vi "LSMcontroller_v58.vi"() -> ()   [LabVIEW 2015] (continued)
                        n3600 = call "waveformsDObuffer.vi"("DO wf in"=w272, "command"="set") -> ()  [unwired: 1 out]
                        n3601 = local write "Total Camera Frames"(w273) -> ()
                        n3602 = local read "wavdet"() -> (w270:bool)
                        n3603 = case shown="True" w270 {
                          tunnel: w269 -> [_ w288]
                          frame False {
                          }
                          frame True {
                            n3604 = local write "# of frames"(w288) -> ()
                          }
                        }
                      }
                    }
                  }
                  frame #6 {
                    w295 = FALSE ("addAO")
                    # "set signaling boolean to false"
                    n3605 = local read "finite samples"() -> (w296:bool)
                    n3606 = local read "continuous"() -> (w297:bool)
                    n3607 = local read "wavdet"() -> (w298:bool)
                    n3608 = call "2pparameters.vi"("command"="get") -> ("params out"=w301:T12)  [unwired: 1 in]
                    n3609 = Bundle By Name(cluster=w301, "finite"=w296, "cont"=w297, "wavdet"=w298) -> (w299:T12)
                    n3610 = local write "addAO"(w295) -> ()
                    n3611 = property on="Add AO wave" class="Bool (strict)"("Val(Sgnl)"=w295) -> ()  [unwired: 2 in, 2 out]
                    n3612 = call "2pparameters.vi"("Params in"=w299, "command"="set") -> ()  [unwired: 1 out]
                  }
                }
              }
            }
          }
          event "AO channels": Value Change {
            n3613 = event-data() -> ()  [unwired: 1 in, 6 out]
            n3614 = local read "AO channels"() -> (w303:u32)
            n3615 = call "2pparameters.vi"("command"="get") -> ("params out"=w305:T12)  [unwired: 1 in]
            n3616 = Unbundle By Name(w305) -> ("aAO"=w304:u32[])
            n3617 = Search 1D Array(1D array=w304, element=w303) -> (index of element=w307:i32)  [unwired: 1 in]
            n3618 = Equal?(x=w307, y=-1.0) -> (x = y?=w308:bool)
            n3619 = case shown="False" w308 {
              tunnel: w307 -> [w310 _]
              frame False {
                n3620 = call "waveformparamsv2.vi"("command"="get") -> ("Params out"=w317:T16)  [unwired: 4 in, 2 out]
                n3621 = Unbundle By Name(w317) -> ("AO parameters"=w316:T17)
                n3622 = Index Array(array=w316, index=w310) -> (element=w333:T18)
                n3623 = Unbundle By Name(w333) -> ("AOtab"=w314:dbl, "Repeats"=w332:dbl, "Cycles"=w331:dbl, "Start amplitude (V)"=w330:dbl, "Baseline (V)"=w329:dbl, "Step size (V)"=w328:dbl, "DC (%)"=w327:dbl, "Sampling frequency (Hz)"=w326:dbl, "Period (ms)"=w325:dbl, "Offset (V)"=w324:dbl, "Amplitude (V)"=w323:dbl, "Frequency"=w322:dbl, "Tri Repeats"=w321:dbl, "phase shift (ms)"=w320:dbl, "Pulses"=w319:dbl, "Tri phase"=w315:dbl, "padding value"=w311:dbl, "Matlab wave file"=w312:path)
                n3624 = To Unsigned Long Integer(number=w314) -> (unsigned 32bit integer=w313:u32)
                n3625 = local write "Build analog waveform tabs"(w313) -> ()
                n3626 = local write "Matlab waveform path"(w312) -> ()
                n3627 = local write "phase shift (ms)"(w320) -> ()
                n3628 = local write "Repeats"(w332) -> ()
                n3629 = local write "Cycles"(w331) -> ()
                n3630 = local write "Amplitude (V)"(w323) -> ()
                n3631 = local write "Matlab padding value"(w311) -> ()
                n3632 = local write "Tri padding value"(w311) -> ()
                n3633 = local write "Start amplitude (V)"(w330) -> ()
                n3634 = local write "Tri Phase (s)"(w315) -> ()
                n3635 = local write "Period (ms)"(w325) -> ()
                n3636 = local write "Tri Repeats"(w321) -> ()
                n3637 = local write "Offset (V)"(w324) -> ()
                n3638 = local write "Frequency"(w322) -> ()
                n3639 = local write "Pulses"(w319) -> ()
                n3640 = local write "padding value"(w311) -> ()
                n3641 = local write "Sampling rate \ncurrent wf"(w326) -> ()
                n3642 = local write "Baseline (V)"(w329) -> ()
                n3643 = local write "Step size (V)"(w328) -> ()
                n3644 = local write "DC (%)"(w327) -> ()
                "Numeric" <- w310
              }
              frame True {
              }
            }
          }
          event "Rem AO wave": Value Change {
            n3645 = event-data() -> ("NewVal"=w334:bool)  [unwired: 1 in, 5 out]
            n3646 = case shown="True" w334 {
              frame False {
              }
              frame True {
                n3647 = stacked-sequence {
                  seq-local: [_ _ w440 _ _ _ _] -> [_ _ _ _ w460 w463 _]
                  frame #0 {
                    n3648 = local read "Measurement"() -> (w335:T5)
                    n3649 = case shown="\"X-Y-t movie\", Default" w335 {
                      frame "X-Y-t movie", Default {
                        n3650 = local read "avpp"() -> (w356:i32)
                        n3651 = local read "Angle ref"() -> (w355:dbl)
                        n3652 = local read "ROI Type"() -> (w354:u16)
                        n3653 = local read "xpixels ref"() -> (w351:i32)
                        n3654 = local read "Vx-min ref"() -> (w350:dbl)
                        n3655 = local read "Vx-max ref"() -> (w349:dbl)
                        n3656 = local read "ypixels ref"() -> (w347:i32)
                        n3657 = local read "Vy-min ref"() -> (w348:dbl)
                        n3658 = local read "Vy-max ref"() -> (w344:dbl)
                        n3659 = local read "Sampling rate"() -> (w338:dbl)
                        n3660 = local read "finite samples"() -> (w339:bool)
                        n3661 = local read "continuous"() -> (w342:bool)
                        n3662 = local read "wavdet"() -> (w343:bool)
                        n3663 = local read "# of frames"() -> (w341:i32)
                        n3664 = local read "maxbufferAI"() -> (w340:i32)
                        n3665 = local read "Override AI buffer"() -> (w336:bool)
                        n3666 = call "2pparameters.vi"("command"="get") -> ("params out"=w353:T12)  [unwired: 1 in]
                        n3667 = Bundle By Name(cluster=w353, "type"="X-Y-t movie", "avpp"=w356, "Angle Img"=w355, "Xpixels Img"=w351, "Vx-min Img"=w350, "VX-max Img"=w349, "Ypixels Img"=w347, "Vy-min Img"=w348, "Vy-max Img"=w344, "srate"=w338, "srate Img"=w338, "finite"=w339, "cont"=w342, "wavdet"=w343, "measpoints"=w341, "maxbufferAI"=w340, "Drawing Mode"=w354, "Vz-reset"=0.0, "AIoverride"=w336) -> (w345:T12)
                        n3668 = call "2pparameters.vi"("Params in"=w345, "command"="set") -> ()  [unwired: 1 out]
                      }
                      frame "X-Y-Z stack" {
                        n3669 = call "2pparameters.vi"("command"="get") -> ("params out"=w360:T12)  [unwired: 1 in]
                        n3670 = Bundle By Name(cluster=w360, "type"="X-Y-Z stack") -> (w358:T12)
                        n3671 = call "2pparameters.vi"("Params in"=w358, "command"="set") -> ()  [unwired: 1 out]
                      }
                      frame "Lifetime (scan)" {
                        n3672 = call "2pparameters.vi"("command"="get") -> ("params out"=w365:T12)  [unwired: 1 in]
                        n3673 = Bundle By Name(cluster=w365, "type"="Lifetime (scan)") -> (w363:T12)
                        n3674 = call "2pparameters.vi"("Params in"=w363, "command"="set") -> ()  [unwired: 1 out]
                      }
                      frame "Lifetime (contour)" {
                        n3675 = local read "Vy-min draw"() -> (w375:dbl)
                        n3676 = local read "Vy-max draw"() -> (w374:dbl)
                        n3677 = local read "Vx-min draw"() -> (w377:dbl)
                        n3678 = local read "Vx-max draw"() -> (w376:dbl)
                        n3679 = local read "xpixels ref"() -> (w373:i32)
                        n3680 = local read "ypixels ref"() -> (w372:i32)
                        n3681 = local read "ROI Type"() -> (w371:u16)
                        n3682 = local read "srateAODOtt"() -> (w382:dbl)
                        n3683 = local read "# of frames"() -> (w387:i32)
                        n3684 = local read "refreshtime"() -> (w379:dbl)
                        n3685 = local read "Pel"() -> (w370:dbl)
                        n3686 = local read "bin"() -> (w385:dbl)
                        n3687 = local read "Override AI buffer"() -> (w368:bool)
                        n3688 = local read "finite samples"() -> (w394:bool)
                        n3689 = local read "srateAODOtt"() -> (w381:dbl)
                        n3690 = local read "srateAODOtt"() -> (w388:dbl)
                        n3691 = local read "continuous"() -> (w393:bool)
                        n3692 = local read "Angle ref"() -> (w378:dbl)
                        n3693 = local read "wavdet"() -> (w395:bool)
                        n3694 = local read "Vx-ref"() -> (w390:dbl)
                        n3695 = local read "Vy-ref"() -> (w392:dbl)
                        n3696 = local read "avpp"() -> (w391:i32)
                        n3697 = call "tt_timeandsamples.vi"("bin"=w385, "refreshtime"=w379, "srateAODOtt"=w382, "tot#ofsamples"=w387) -> ("refreshrate"=w383:dbl, "refreshbuffer"=w384:i32, "timetracecycles"=w389:i32)  [unwired: 5 in]
                        n3698 = local read "bin"() -> (w386:dbl)
                        n3699 = call "2pparameters.vi"("command"="get") -> ("params out"=w398:T12)  [unwired: 1 in]
                        n3700 = Bundle By Name(cluster=w398, "Drawing Mode"=w371, "measpoints"=w387, "tt_cycles"=w389, "refreshbuffer"=w384, "refreshrate"=w383, "Vx-ref"=w390, "Vy-ref"=w392, "srate"=w381, "finite"=w394, "cont"=w393, "wavdet"=w395, "avpp"=w391, "srateAODO"=w388, "bufferAI"=w384, "bin"=w386, "Angle Img"=w378, "Vxminref"=w377, "Vxmaxref"=w376, "Vyminref"=w375, "Vymaxref"=w374, "Xpixels Img"=w373, "Ypixels Img"=w372, "Pel"=w370, "Vz-reset"=0.0, "AIoverride"=w368, "type"="Lifetime (contour)") -> (w396:T12)
                        n3701 = Reciprocal(x=w383) -> (1/x=w380:dbl)
                        n3702 = local write "refreshtime"(w380) -> ()
                        n3703 = call "2pparameters.vi"("Params in"=w396, "command"="set") -> ()  [unwired: 1 out]
                      }
                      frame "X-Y-Z-t movie" {
                      }
                      frame "linescan" {
                      }
                      frame "Timetrace" {
                        n3704 = local read "Vy-min draw"() -> (w408:dbl)
                        n3705 = local read "Vy-max draw"() -> (w407:dbl)
                        n3706 = local read "Vx-min draw"() -> (w410:dbl)
                        n3707 = local read "Vx-max draw"() -> (w409:dbl)
                        n3708 = local read "xpixels ref"() -> (w406:i32)
                        n3709 = local read "ypixels ref"() -> (w405:i32)
                        n3710 = local read "ROI Type"() -> (w404:u16)
                        n3711 = local read "srateAODOtt"() -> (w415:dbl)
                        n3712 = local read "# of frames"() -> (w420:i32)
                        n3713 = local read "refreshtime"() -> (w412:dbl)
                        n3714 = local read "Pel"() -> (w403:dbl)
                        n3715 = local read "bin"() -> (w418:dbl)
                        n3716 = local read "Override AI buffer"() -> (w401:bool)
                        n3717 = local read "finite samples"() -> (w427:bool)
                        n3718 = local read "srateAODOtt"() -> (w414:dbl)
                        n3719 = local read "srateAODOtt"() -> (w421:dbl)
                        n3720 = local read "continuous"() -> (w426:bool)
                        n3721 = local read "Angle ref"() -> (w411:dbl)
                        n3722 = local read "wavdet"() -> (w428:bool)
                        n3723 = local read "Vx-ref"() -> (w423:dbl)
                        n3724 = local read "Vy-ref"() -> (w425:dbl)
                        n3725 = local read "avpp"() -> (w424:i32)
                        n3726 = call "tt_timeandsamples.vi"("bin"=w418, "refreshtime"=w412, "srateAODOtt"=w415, "tot#ofsamples"=w420) -> ("refreshrate"=w416:dbl, "refreshbuffer"=w417:i32, "timetracecycles"=w422:i32)  [unwired: 5 in]
                        n3727 = local read "bin"() -> (w419:dbl)
                        n3728 = call "2pparameters.vi"("command"="get") -> ("params out"=w431:T12)  [unwired: 1 in]
                        n3729 = Bundle By Name(cluster=w431, "Drawing Mode"=w404, "measpoints"=w420, "tt_cycles"=w422, "refreshbuffer"=w417, "refreshrate"=w416, "Vx-ref"=w423, "Vy-ref"=w425, "srate"=w414, "finite"=w427, "cont"=w426, "wavdet"=w428, "avpp"=w424, "srateAODO"=w421, "bufferAI"=w417, "bin"=w419, "Angle Img"=w411, "Vxminref"=w410, "Vxmaxref"=w409, "Vyminref"=w408, "Vymaxref"=w407, "Xpixels Img"=w406, "Ypixels Img"=w405, "Pel"=w403, "Vz-reset"=0.0, "AIoverride"=w401, "type"="Timetrace") -> (w429:T12)
                        n3730 = Reciprocal(x=w416) -> (1/x=w413:dbl)
                        n3731 = local write "refreshtime"(w413) -> ()
                        n3732 = call "2pparameters.vi"("Params in"=w429, "command"="set") -> ()  [unwired: 1 out]
                      }
                      frame "Lifetime (point)" {
                      }
                    }
                  }
                  frame #1 {
                    w434 = FALSE ("wavdet")
                    n3733 = call "2pparameters.vi"("command"="get") -> ("params out"=w438:T12)  [unwired: 1 in]
                    n3734 = Bundle By Name(cluster=w438, "finite"=w434, "cont"=w434, "wavdet"=TRUE) -> (w435:T12)
                    n3735 = call "2pparameters.vi"("Params in"=w435, "command"="set") -> ()  [unwired: 1 out]
                  }
                  frame #2 {
                    # "remove channel from numbers array"
                    n3736 = local read "AO channels"() -> (w445:u32)
                    n3737 = call "2pparameters.vi"("command"="get") -> ("params out"=w443:T12)  [unwired: 1 in]
                    n3738 = in-place {
                      in-place-border: w445 -> [w451]
                      in-place-border: [w448] -> w446
                      in-place-border: [w447] -> w440
                      n3739 = in-place-cluster #50(w443) -> ("aAO"=w450:u32[])
                      n3740 = call "remove channel from active arrayv2.vi"("line array in"=w450, "line to remove"=w451) -> ("line array out"=w449:u32[], "removal"=w448:bool, "index"=w447:i32)
                      n3741 = in-place-cluster #50("aAO"=w449) -> (w441:T12)
                    }
                    n3742 = local write "remAO"(w446) -> ()
                    n3743 = call "2pparameters.vi"("Params in"=w441, "command"="set") -> ()  [unwired: 1 out]
                  }
                  frame #3 {
                    n3744 = local read "remAO"() -> (w452:bool)
                    n3745 = case shown="True" w452 {
                      frame False {
                      }
                      frame True {
                        n3746 = call "Used AO lines.vi"() -> ("used AO names"=w456:string[], "used AO lines"=w458:tag[])  [unwired: 2 in]
                        n3747 = control-ref of="Analog Lines Plot"() -> (w457:refnum<vi>)
                        n3748 = control-ref of="Digital Lines Plot"() -> (w455:refnum<vi>)
                        n3749 = call "Used DO lines.vi"() -> ("used DO names"=w454:string[], "used DO lines"=w453:tag[])  [unwired: 2 in]
                        n3750 = local write "Analog Used Lines"(w458) -> ()
                        n3751 = local write "Analog Used Names"(w456) -> ()
                        n3752 = local write "Digital Used Lines"(w453) -> ()
                        n3753 = local write "Digital Used Names"(w454) -> ()
                        n3754 = call "prepDOWaveplot.vi"("DigitalGraph in"=w455, "used DO names"=w454) -> ()  [unwired: 1 in]
                        n3755 = call "prepAOWaveplot.vi"("WaveformGraph in"=w457, "Analog Used Names"=w456) -> ()  [unwired: 1 in]
                      }
                    }
                  }
                  frame #4 {
                    n3756 = local read "remAO"() -> (w459:bool)
                    n3757 = case shown="True" w459 {
                      tunnel: w460 -> [_ w461]
                      frame False {
                      }
                      frame True {
                        n3758 = call "waveformparamsv2.vi"("command"="rem AO", "index"=w461) -> ()  [unwired: 3 in, 3 out]
                      }
                    }
                  }
                  frame #5 {
                    n3759 = local read "remAO"() -> (w464:bool)
                    n3760 = case shown="True" w464 {
                      tunnel: w463 -> [_ w483]
                      frame False {
                      }
                      frame True {
                        n3761 = local read "Meastab"() -> (w468:enum32{"X-Y Image", "Linescan", "Timetrace"})
                        n3762 = property on="refwf" class="Ring (strict)"() -> ("RingText.Text"=w471:string)  [unwired: 2 in, 2 out]
                        n3763 = case shown="\"Timetrace\"" w468 {
                          tunnel: [w484 w485] -> w467
                          frame "X-Y Image", Default {
                            n3764 = local read "Sampling rate"() -> (w484:dbl)
                          }
                          frame "Timetrace" {
                            n3765 = local read "srateAODOtt"() -> (w485:dbl)
                          }
                        }
                        n3766 = call "waveformsAObuffer.vi"("command"="get") -> ("AO wf out"=w480:waveform(dbl)[])  [unwired: 1 in]
                        n3767 = call "waveformsDObuffer.vi"("command"="get") -> ("DO wf out"=w477:digitalwaveform[])  [unwired: 1 in]
                        n3768 = Delete From Array(array=w480, length=1, index=w483) -> (array with subset deleted=w472:waveform(dbl)[])  [unwired: 1 out]
                        n3769 = call "correctwaveformsizetemp.vi"("new sampling frequency (Hz)"=w467, "start"=FALSE, "reference waveforms to"=w471, "Analog waveforms in"=w472, "stop"=FALSE, "Digital waveforms in"=w477) -> ("analog wf out"=w475:waveform(dbl)[], "Digital wf out"=w473:digitalwaveform[], "measpoints"=w469:i32)
                        n3770 = local write "Analog Lines Plot"(w475) -> ()
                        n3771 = call "GetNumCamFramesv2.vi"("Digital Waveform Graph"=w473) -> ("Numeric"=w474:i32)  [unwired: 10 in]
                        n3772 = local write "Digital Lines Plot"(w473) -> ()
                        n3773 = call "waveformsAObuffer.vi"("AO wf in"=w475, "command"="set") -> ()  [unwired: 1 out]
                        n3774 = call "waveformsDObuffer.vi"("DO wf in"=w473, "command"="set") -> ()  [unwired: 1 out]
                        n3775 = local read "wavdet"() -> (w470:bool)
                        n3776 = local write "Total Camera Frames"(w474) -> ()
                        n3777 = case shown="True" w470 {
                          tunnel: w469 -> [_ w486]
                          frame False {
                          }
                          frame True {
                            n3778 = local write "# of frames"(w486) -> ()
                          }
                        }
                      }
                    }
                  }
                  frame #6 {
                    w487 = FALSE ("remAO")
                    n3779 = local read "finite samples"() -> (w488:bool)
                    n3780 = local read "continuous"() -> (w489:bool)
                    n3781 = local read "wavdet"() -> (w490:bool)
                    n3782 = call "2pparameters.vi"("command"="get") -> ("params out"=w493:T12)  [unwired: 1 in]
                    n3783 = Bundle By Name(cluster=w493, "finite"=w488, "cont"=w489, "wavdet"=w490) -> (w491:T12)
                    n3784 = local write "remAO"(w487) -> ()
                    n3785 = property on="Rem AO wave" class="Bool (strict)"("Val(Sgnl)"=w487) -> ()  [unwired: 2 in, 2 out]
                    n3786 = call "2pparameters.vi"("Params in"=w491, "command"="set") -> ()  [unwired: 1 out]
                  }
                }
              }
            }
          }
          event "Add DO wave": Value Change {
            n3787 = event-data() -> ("NewVal"=w495:bool)  [unwired: 1 in, 5 out]
            n3788 = case shown="True" w495 {
              frame False {
              }
              frame True {
                n3789 = stacked-sequence {
                  seq-local: [_ _ _ _ _ w655 _ _] -> [_ _ _ _ _ _ w670 _]
                  frame #0 {
                    n3790 = local read "Measurement"() -> (w496:T5)
                    n3791 = case shown="\"X-Y-t movie\", Default" w496 {
                      frame "X-Y-t movie", Default {
                        n3792 = local read "avpp"() -> (w517:i32)
                        n3793 = local read "Angle ref"() -> (w516:dbl)
                        n3794 = local read "ROI Type"() -> (w515:u16)
                        n3795 = local read "xpixels ref"() -> (w512:i32)
                        n3796 = local read "Vx-min ref"() -> (w511:dbl)
                        n3797 = local read "Vx-max ref"() -> (w510:dbl)
                        n3798 = local read "ypixels ref"() -> (w508:i32)
                        n3799 = local read "Vy-min ref"() -> (w509:dbl)
                        n3800 = local read "Vy-max ref"() -> (w505:dbl)
                        n3801 = local read "Sampling rate"() -> (w499:dbl)
                        n3802 = local read "finite samples"() -> (w500:bool)
                        n3803 = local read "continuous"() -> (w503:bool)
                        n3804 = local read "wavdet"() -> (w504:bool)
                        n3805 = local read "# of frames"() -> (w502:i32)
                        n3806 = local read "maxbufferAI"() -> (w501:i32)
                        n3807 = local read "Override AI buffer"() -> (w497:bool)
                        n3808 = call "2pparameters.vi"("command"="get") -> ("params out"=w514:T12)  [unwired: 1 in]
                        n3809 = Bundle By Name(cluster=w514, "type"="X-Y-t movie", "avpp"=w517, "Angle Img"=w516, "Xpixels Img"=w512, "Vx-min Img"=w511, "VX-max Img"=w510, "Ypixels Img"=w508, "Vy-min Img"=w509, "Vy-max Img"=w505, "srate"=w499, "srate Img"=w499, "finite"=w500, "cont"=w503, "wavdet"=w504, "measpoints"=w502, "maxbufferAI"=w501, "Drawing Mode"=w515, "Vz-reset"=0.0, "AIoverride"=w497) -> (w506:T12)
                        n3810 = call "2pparameters.vi"("Params in"=w506, "command"="set") -> ()  [unwired: 1 out]
                      }
                      frame "X-Y-Z stack" {
                        n3811 = call "2pparameters.vi"("command"="get") -> ("params out"=w521:T12)  [unwired: 1 in]
                        n3812 = Bundle By Name(cluster=w521, "type"="X-Y-Z stack") -> (w519:T12)
                        n3813 = call "2pparameters.vi"("Params in"=w519, "command"="set") -> ()  [unwired: 1 out]
                      }
                      frame "Lifetime (scan)" {
                        n3814 = call "2pparameters.vi"("command"="get") -> ("params out"=w526:T12)  [unwired: 1 in]
                        n3815 = Bundle By Name(cluster=w526, "type"="Lifetime (scan)") -> (w524:T12)
                        n3816 = call "2pparameters.vi"("Params in"=w524, "command"="set") -> ()  [unwired: 1 out]
                      }
                      frame "Lifetime (contour)" {
                        n3817 = local read "Vy-min draw"() -> (w536:dbl)
                        n3818 = local read "Vy-max draw"() -> (w535:dbl)
                        n3819 = local read "Vx-min draw"() -> (w538:dbl)
                        n3820 = local read "Vx-max draw"() -> (w537:dbl)
                        n3821 = local read "xpixels ref"() -> (w534:i32)
                        n3822 = local read "ypixels ref"() -> (w533:i32)
                        n3823 = local read "ROI Type"() -> (w532:u16)
                        n3824 = local read "srateAODOtt"() -> (w543:dbl)
                        n3825 = local read "# of frames"() -> (w548:i32)
                        n3826 = local read "refreshtime"() -> (w540:dbl)
                        n3827 = local read "Pel"() -> (w531:dbl)
                        n3828 = local read "bin"() -> (w546:dbl)
                        n3829 = local read "Override AI buffer"() -> (w529:bool)
                        n3830 = local read "finite samples"() -> (w555:bool)
                        n3831 = local read "srateAODOtt"() -> (w542:dbl)
                        n3832 = local read "srateAODOtt"() -> (w549:dbl)
                        n3833 = local read "continuous"() -> (w554:bool)
                        n3834 = local read "Angle ref"() -> (w539:dbl)
                        n3835 = local read "wavdet"() -> (w556:bool)
                        n3836 = local read "Vx-ref"() -> (w551:dbl)
                        n3837 = local read "Vy-ref"() -> (w553:dbl)
                        n3838 = local read "avpp"() -> (w552:i32)
                        n3839 = call "tt_timeandsamples.vi"("bin"=w546, "refreshtime"=w540, "srateAODOtt"=w543, "tot#ofsamples"=w548) -> ("refreshrate"=w544:dbl, "refreshbuffer"=w545:i32, "timetracecycles"=w550:i32)  [unwired: 5 in]
                        n3840 = local read "bin"() -> (w547:dbl)
                        n3841 = call "2pparameters.vi"("command"="get") -> ("params out"=w559:T12)  [unwired: 1 in]
                        n3842 = Bundle By Name(cluster=w559, "Drawing Mode"=w532, "measpoints"=w548, "tt_cycles"=w550, "refreshbuffer"=w545, "refreshrate"=w544, "Vx-ref"=w551, "Vy-ref"=w553, "srate"=w542, "finite"=w555, "cont"=w554, "wavdet"=w556, "avpp"=w552, "srateAODO"=w549, "bufferAI"=w545, "bin"=w547, "Angle Img"=w539, "Vxminref"=w538, "Vxmaxref"=w537, "Vyminref"=w536, "Vymaxref"=w535, "Xpixels Img"=w534, "Ypixels Img"=w533, "Pel"=w531, "Vz-reset"=0.0, "AIoverride"=w529, "type"="Lifetime (contour)") -> (w557:T12)
                        n3843 = Reciprocal(x=w544) -> (1/x=w541:dbl)
                        n3844 = local write "refreshtime"(w541) -> ()
                        n3845 = call "2pparameters.vi"("Params in"=w557, "command"="set") -> ()  [unwired: 1 out]
                      }
                      frame "X-Y-Z-t movie" {
                      }
                      frame "linescan" {
                      }
                      frame "Timetrace" {
                        n3846 = local read "Vy-min draw"() -> (w569:dbl)
                        n3847 = local read "Vy-max draw"() -> (w568:dbl)
                        n3848 = local read "Vx-min draw"() -> (w571:dbl)
                        n3849 = local read "Vx-max draw"() -> (w570:dbl)
                        n3850 = local read "xpixels ref"() -> (w567:i32)
                        n3851 = local read "ypixels ref"() -> (w566:i32)
                        n3852 = local read "ROI Type"() -> (w565:u16)
                        n3853 = local read "srateAODOtt"() -> (w576:dbl)
                        n3854 = local read "# of frames"() -> (w581:i32)
                        n3855 = local read "refreshtime"() -> (w573:dbl)
                        n3856 = local read "Pel"() -> (w564:dbl)
                        n3857 = local read "bin"() -> (w579:dbl)
                        n3858 = local read "Override AI buffer"() -> (w562:bool)
                        n3859 = local read "finite samples"() -> (w588:bool)
                        n3860 = local read "srateAODOtt"() -> (w575:dbl)
                        n3861 = local read "srateAODOtt"() -> (w582:dbl)
                        n3862 = local read "continuous"() -> (w587:bool)
                        n3863 = local read "Angle ref"() -> (w572:dbl)
                        n3864 = local read "wavdet"() -> (w589:bool)
                        n3865 = local read "Vx-ref"() -> (w584:dbl)
                        n3866 = local read "Vy-ref"() -> (w586:dbl)
                        n3867 = local read "avpp"() -> (w585:i32)
                        n3868 = call "tt_timeandsamples.vi"("bin"=w579, "refreshtime"=w573, "srateAODOtt"=w576, "tot#ofsamples"=w581) -> ("refreshrate"=w577:dbl, "refreshbuffer"=w578:i32, "timetracecycles"=w583:i32)  [unwired: 5 in]
                        n3869 = local read "bin"() -> (w580:dbl)
                        n3870 = call "2pparameters.vi"("command"="get") -> ("params out"=w592:T12)  [unwired: 1 in]
                        n3871 = Bundle By Name(cluster=w592, "Drawing Mode"=w565, "measpoints"=w581, "tt_cycles"=w583, "refreshbuffer"=w578, "refreshrate"=w577, "Vx-ref"=w584, "Vy-ref"=w586, "srate"=w575, "finite"=w588, "cont"=w587, "wavdet"=w589, "avpp"=w585, "srateAODO"=w582, "bufferAI"=w578, "bin"=w580, "Angle Img"=w572, "Vxminref"=w571, "Vxmaxref"=w570, "Vyminref"=w569, "Vymaxref"=w568, "Xpixels Img"=w567, "Ypixels Img"=w566, "Pel"=w564, "Vz-reset"=0.0, "AIoverride"=w562, "type"="Timetrace") -> (w590:T12)
                        n3872 = Reciprocal(x=w577) -> (1/x=w574:dbl)
                        n3873 = local write "refreshtime"(w574) -> ()
                        n3874 = call "2pparameters.vi"("Params in"=w590, "command"="set") -> ()  [unwired: 1 out]
                      }
                      frame "Lifetime (point)" {
                      }
                    }
                  }
                  frame #1 {
                    w595 = FALSE ("wavdet")
                    n3875 = call "2pparameters.vi"("command"="get") -> ("params out"=w599:T12)  [unwired: 1 in]
                    n3876 = Bundle By Name(cluster=w599, "finite"=w595, "cont"=w595, "wavdet"=TRUE) -> (w596:T12)
                    n3877 = call "2pparameters.vi"("Params in"=w596, "command"="set") -> ()  [unwired: 1 out]
                  }
                  frame #2 {
                    n3878 = local read "DO channels"() -> (w606:u16)
                    n3879 = call "2pparameters.vi"("command"="get") -> ("params out"=w604:T12)  [unwired: 1 in]
                    n3880 = in-place {
                      in-place-border: w606 -> [w610]
                      in-place-border: [w607] -> w601
                      n3881 = in-place-cluster #51(w604) -> ("aDO"=w609:u32[])
                      n3882 = call "add channel to active arrayv2.vi"("line array in"=w609, "line to add"=w610) -> ("line array out"=w608:u32[], "addition"=w607:bool)  [unwired: 1 out]
                      n3883 = in-place-cluster #51("aDO"=w608) -> (w602:T12)
                    }
                    n3884 = local write "addDO"(w601) -> ()
                    n3885 = call "2pparameters.vi"("Params in"=w602, "command"="set") -> ()  [unwired: 1 out]
                  }
                  frame #3 {
                    n3886 = local read "addDO"() -> (w611:bool)
                    n3887 = case shown="True" w611 {
                      frame False {
                      }
                      frame True {
                        n3888 = call "Used AO lines.vi"() -> ("used AO names"=w615:string[], "used AO lines"=w617:tag[])  [unwired: 2 in]
                        n3889 = control-ref of="Analog Lines Plot"() -> (w616:refnum<vi>)
                        n3890 = control-ref of="Digital Lines Plot"() -> (w614:refnum<vi>)
                        n3891 = call "Used DO lines.vi"() -> ("used DO names"=w613:string[], "used DO lines"=w612:tag[])  [unwired: 2 in]
                        n3892 = local write "Analog Used Lines"(w617) -> ()
                        n3893 = local write "Analog Used Names"(w615) -> ()
                        n3894 = local write "Digital Used Lines"(w612) -> ()
                        n3895 = local write "Digital Used Names"(w613) -> ()
                        n3896 = call "prepDOWaveplot.vi"("DigitalGraph in"=w614, "used DO names"=w613) -> ()  [unwired: 1 in]
                        n3897 = call "prepAOWaveplot.vi"("WaveformGraph in"=w616, "Analog Used Names"=w615) -> ()  [unwired: 1 in]
                      }
                    }
                  }
                  frame #4 {
                    n3898 = local read "addDO"() -> (w618:bool)
                    n3899 = case shown="True" w618 {
                      frame False {
                      }
                      frame True {
                        n3900 = local read "Build digital waveform tabs"() -> (w619:enum32{"Simple", "Matlab"})
                        n3901 = case shown="\"Matlab\"" w619 {
                          frame "Simple", Default {
                            n3902 = local read "Meastab"() -> (w621:enum32{"X-Y Image", "Linescan", "Timetrace"})
                            n3903 = call "waveformparamsv2.vi"("command"="get") -> ("Params out"=w635:T16)  [unwired: 4 in, 2 out]
                            n3904 = case shown="\"Timetrace\"" w621 {
                              tunnel: [w637 w638] -> w620
                              frame "X-Y Image", Default {
                                n3905 = local read "Sampling rate"() -> (w637:dbl)
                              }
                              frame "Timetrace" {
                                n3906 = local read "srateAODOtt"() -> (w638:dbl)
                              }
                            }
                            n3907 = Unbundle By Name(w635) -> ("DO parameters"=w633:T19)
                            n3908 = local read "Digital padding value"() -> (w624:dbl)
                            n3909 = local read "Digital time offset (s)"() -> (w625:dbl)
                            n3910 = local read "Digital phase (s)"() -> (w627:dbl)
                            n3911 = local read "Digital Freq (Hz)"() -> (w626:dbl)
                            n3912 = local read "Digital DC (%)"() -> (w628:dbl)
                            n3913 = Index Array(array=w633, index=0) -> (element=w632:T20)
                            n3914 = Bundle By Name(cluster=w632, "Digital DC (%)"=w628, "Digital phase"=w627, "Digital Freq (Hz)"=w626, "Sampling frequency (Hz)"=w620, "Digital time offset (s)"=w625, "padding value"=w624, "matlab wave file"=path "", "DOtab"=0.0) -> (w630:T20)
                            n3915 = Build Array(w630) -> (w629:T19)
                            n3916 = call "waveformparamsv2.vi"("command"="add DO", "add DO"=w629) -> ()  [unwired: 3 in, 3 out]
                          }
                          frame "Matlab" {
                            w642 = 0.0 ("DOtab")
                            n3917 = local read "Meastab"() -> (w640:enum32{"X-Y Image", "Linescan", "Timetrace"})
                            n3918 = call "waveformparamsv2.vi"("command"="get") -> ("Params out"=w651:T16)  [unwired: 4 in, 2 out]
                            n3919 = case shown="\"Timetrace\"" w640 {
                              tunnel: [w653 w654] -> w639
                              frame "X-Y Image", Default {
                                n3920 = local read "Sampling rate"() -> (w653:dbl)
                              }
                              frame "Timetrace" {
                                n3921 = local read "srateAODOtt"() -> (w654:dbl)
                              }
                            }
                            n3922 = Unbundle By Name(w651) -> ("DO parameters"=w649:T19)
                            n3923 = local read "Matlab waveform path DO"() -> (w641:path)
                            n3924 = local read "Matlab padding value DO"() -> (w644:dbl)
                            n3925 = Index Array(array=w649, index=0) -> (element=w648:T20)
                            n3926 = Bundle By Name(cluster=w648, "Digital DC (%)"=w642, "Digital phase"=w642, "Digital Freq (Hz)"=w642, "Sampling frequency (Hz)"=w639, "Digital time offset (s)"=w642, "padding value"=w644, "matlab wave file"=w641, "DOtab"=1.0) -> (w646:T20)
                            n3927 = Build Array(w646) -> (w645:T19)
                            n3928 = call "waveformparamsv2.vi"("command"="add DO", "add DO"=w645) -> ()  [unwired: 3 in, 3 out]
                          }
                        }
                      }
                    }
                  }
                  frame #5 {
                    n3929 = local read "addDO"() -> (w656:bool)
                    n3930 = case shown="True" w656 {
                      tunnel: [_ w657] -> w655
                      frame False {
                      }
                      frame True {
                        n3931 = property on="refwf" class="Ring (strict)"() -> ("RingText.Text"=w662:string)  [unwired: 2 in, 2 out]
                        n3932 = call "waveformsDObuffer.vi"("command"="get") -> ("DO wf out"=w661:digitalwaveform[])  [unwired: 1 in]
                        n3933 = call "waveformsAObuffer.vi"("command"="get") -> ("AO wf out"=w659:waveform(dbl)[])  [unwired: 1 in]
                        n3934 = call "referfencesize.vi"("Digital waveforms in"=w661, "Analog waveforms in"=w659, "reference waveforms to"=w662) -> ("number of samples"=w657:i32)  [unwired: 2 in]
                      }
                    }
                  }
                  frame #6 {
                    n3935 = local read "Build digital waveform tabs"() -> (w673:enum32{"Simple", "Matlab"})
                    n3936 = call "waveformparamsv2.vi"("command"="get last DO") -> ("last DO"=w672:T20)  [unwired: 4 in, 2 out]
                    n3937 = local read "Meastab"() -> (w666:enum32{"X-Y Image", "Linescan", "Timetrace"})
                    n3938 = call "waveformsDObuffer.vi"("command"="get") -> ("DO wf out"=w671:digitalwaveform[])  [unwired: 1 in]
                    n3939 = case shown="\"Simple\", Default" w673 {
                      tunnel: w672 -> [w690 w692]
                      tunnel: w670 -> [w689 _]
                      tunnel: [w688 w691] -> w669
                      frame "Simple", Default {
                        n3940 = call "simple digital from wf params.vi"("waveform params"=w690, "number of samples"=w689) -> ("digital waveform"=w688:digitalwaveform)
                      }
                      frame "Matlab" {
                        n3941 = call "matlabDOwffromparam.vi"("waveform params"=w692) -> ("digital waveform"=w691:digitalwaveform)
                      }
                    }
                    n3942 = property on="refwf" class="Ring (strict)"() -> ("RingText.Text"=w676:string)  [unwired: 2 in, 2 out]
                    n3943 = case shown="\"Timetrace\"" w666 {
                      tunnel: [w685 w686] -> w665
                      frame "X-Y Image", Default {
                        n3944 = local read "Sampling rate"() -> (w685:dbl)
                      }
                      frame "Timetrace" {
                        n3945 = local read "srateAODOtt"() -> (w686:dbl)
                      }
                    }
                    n3946 = call "waveformsAObuffer.vi"("command"="get") -> ("AO wf out"=w684:waveform(dbl)[])  [unwired: 1 in]
                    n3947 = Build Array (concatenate)(w671, w669) -> (w675:digitalwaveform[])
                    n3948 = call "correctwaveformsizetemp.vi"("new sampling frequency (Hz)"=w665, "start"=FALSE, "reference waveforms to"=w676, "Analog waveforms in"=w684, "stop"=FALSE, "Digital waveforms in"=w675) -> ("analog wf out"=w679:waveform(dbl)[], "Digital wf out"=w677:digitalwaveform[], "measpoints"=w667:i32)
                    n3949 = local write "Analog Lines Plot"(w679) -> ()
                    n3950 = call "GetNumCamFramesv2.vi"("Digital Waveform Graph"=w677) -> ("Numeric"=w678:i32)  [unwired: 10 in]
                    n3951 = local write "Digital Lines Plot"(w677) -> ()
                    n3952 = call "waveformsAObuffer.vi"("AO wf in"=w679, "command"="set") -> ()  [unwired: 1 out]
                    n3953 = call "waveformsDObuffer.vi"("DO wf in"=w677, "command"="set") -> ()  [unwired: 1 out]
                    n3954 = local write "Total Camera Frames"(w678) -> ()
                    n3955 = local read "wavdet"() -> (w668:bool)
                    n3956 = case shown="True" w668 {
                      tunnel: w667 -> [_ w687]
                      frame False {
                      }
                      frame True {
                        n3957 = local write "# of frames"(w687) -> ()
                      }
                    }
                  }
                  frame #7 {
                    w693 = FALSE ("addAO")
                    n3958 = local read "finite samples"() -> (w694:bool)
                    n3959 = local read "continuous"() -> (w695:bool)
                    n3960 = local read "wavdet"() -> (w696:bool)
                    n3961 = call "2pparameters.vi"("command"="get") -> ("params out"=w699:T12)  [unwired: 1 in]
                    n3962 = Bundle By Name(cluster=w699, "finite"=w694, "cont"=w695, "wavdet"=w696) -> (w697:T12)
                    n3963 = call "2pparameters.vi"("Params in"=w697, "command"="set") -> ()  [unwired: 1 out]
                    n3964 = local write "addDO"(w693) -> ()
                    n3965 = property on="Add DO wave" class="Bool (strict)"("Val(Sgnl)"=w693) -> ()  [unwired: 2 in, 2 out]
                  }
                }
              }
            }
          }
          event "DO channels": Value Change {
            n3966 = event-data() -> ()  [unwired: 1 in, 6 out]
            n3967 = local read "DO channels"() -> (w703:u16)
            n3968 = call "2pparameters.vi"("command"="get") -> ("params out"=w705:T12)  [unwired: 1 in]
            n3969 = Unbundle By Name(w705) -> ("aDO"=w704:u32[])
            n3970 = Search 1D Array(1D array=w704, element=w703) -> (index of element=w702:i32)  [unwired: 1 in]
            n3971 = Equal?(x=w702, y=-1.0) -> (x = y?=w701:bool)
            n3972 = case shown="False" w701 {
              tunnel: w702 -> [w720 _]
              frame False {
                n3973 = call "waveformparamsv2.vi"("command"="get") -> ("Params out"=w715:T16)  [unwired: 4 in, 2 out]
                n3974 = Unbundle By Name(w715) -> ("DO parameters"=w713:T19)
                n3975 = Index Array(array=w713, index=w720) -> (element=w719:T20)
                n3976 = Unbundle By Name(w719) -> ("Digital DC (%)"=w718:dbl, "Digital phase"=w717:dbl, "Digital Freq (Hz)"=w716:dbl, "Sampling frequency (Hz)"=w708:dbl, "Digital time offset (s)"=w712:dbl, "padding value"=w711:dbl, "matlab wave file"=w710:path, "DOtab"=w709:dbl)
                n3977 = local write "Build digital waveform tabs"(w709) -> ()
                n3978 = local write "Digital DC (%)"(w718) -> ()
                n3979 = local write "Matlab waveform path DO"(w710) -> ()
                n3980 = local write "Digital time offset (s)"(w712) -> ()
                n3981 = local write "Matlab padding value DO"(w711) -> ()
                n3982 = local write "Digital padding value"(w711) -> ()
                n3983 = local write "Sampling rate \ncurrent wf"(w708) -> ()
                n3984 = local write "Digital Freq (Hz)"(w716) -> ()
                n3985 = local write "Digital phase (s)"(w717) -> ()
              }
              frame True {
              }
            }
          }
          event "Rem DO wave": Value Change {
            n3986 = event-data() -> ("NewVal"=w721:bool)  [unwired: 1 in, 5 out]
            n3987 = case shown="True" w721 {
              frame False {
              }
              frame True {
                n3988 = stacked-sequence {
                  seq-local: [_ _ w827 _ _ _ _] -> [_ _ _ _ w846 w857 _]
                  frame #0 {
                    n3989 = local read "Measurement"() -> (w722:T5)
                    n3990 = case shown="\"linescan\"" w722 {
                      frame "X-Y-t movie", Default {
                        n3991 = local read "avpp"() -> (w743:i32)
                        n3992 = local read "Angle ref"() -> (w742:dbl)
                        n3993 = local read "ROI Type"() -> (w741:u16)
                        n3994 = local read "xpixels ref"() -> (w738:i32)
                        n3995 = local read "Vx-min ref"() -> (w737:dbl)
                        n3996 = local read "Vx-max ref"() -> (w736:dbl)
                        n3997 = local read "ypixels ref"() -> (w734:i32)
                        n3998 = local read "Vy-min ref"() -> (w735:dbl)
                        n3999 = local read "Vy-max ref"() -> (w731:dbl)
                        n4000 = local read "Sampling rate"() -> (w725:dbl)
                        n4001 = local read "finite samples"() -> (w726:bool)
                        n4002 = local read "continuous"() -> (w729:bool)
                        n4003 = local read "wavdet"() -> (w730:bool)
                        n4004 = local read "# of frames"() -> (w728:i32)
                        n4005 = local read "maxbufferAI"() -> (w727:i32)
                        n4006 = local read "Override AI buffer"() -> (w723:bool)
                        n4007 = call "2pparameters.vi"("command"="get") -> ("params out"=w740:T12)  [unwired: 1 in]
                        n4008 = Bundle By Name(cluster=w740, "type"="X-Y-t movie", "avpp"=w743, "Angle Img"=w742, "Xpixels Img"=w738, "Vx-min Img"=w737, "VX-max Img"=w736, "Ypixels Img"=w734, "Vy-min Img"=w735, "Vy-max Img"=w731, "srate"=w725, "srate Img"=w725, "finite"=w726, "cont"=w729, "wavdet"=w730, "measpoints"=w728, "maxbufferAI"=w727, "Drawing Mode"=w741, "Vz-reset"=0.0, "AIoverride"=w723) -> (w732:T12)
                        n4009 = call "2pparameters.vi"("Params in"=w732, "command"="set") -> ()  [unwired: 1 out]
                      }
                      frame "X-Y-Z stack" {
                        n4010 = call "2pparameters.vi"("command"="get") -> ("params out"=w747:T12)  [unwired: 1 in]
                        n4011 = Bundle By Name(cluster=w747, "type"="X-Y-Z stack") -> (w745:T12)
                        n4012 = call "2pparameters.vi"("Params in"=w745, "command"="set") -> ()  [unwired: 1 out]
                      }
                      frame "Lifetime (scan)" {
                        n4013 = call "2pparameters.vi"("command"="get") -> ("params out"=w752:T12)  [unwired: 1 in]
                        n4014 = Bundle By Name(cluster=w752, "type"="Lifetime (scan)") -> (w750:T12)
                        n4015 = call "2pparameters.vi"("Params in"=w750, "command"="set") -> ()  [unwired: 1 out]
                      }
                      frame "Lifetime (contour)" {
                        n4016 = local read "Vy-min draw"() -> (w762:dbl)
                        n4017 = local read "Vy-max draw"() -> (w761:dbl)
                        n4018 = local read "Vx-min draw"() -> (w764:dbl)
                        n4019 = local read "Vx-max draw"() -> (w763:dbl)
                        n4020 = local read "xpixels ref"() -> (w760:i32)
                        n4021 = local read "ypixels ref"() -> (w759:i32)
                        n4022 = local read "ROI Type"() -> (w758:u16)
                        n4023 = local read "srateAODOtt"() -> (w769:dbl)
                        n4024 = local read "# of frames"() -> (w774:i32)
                        n4025 = local read "refreshtime"() -> (w766:dbl)
                        n4026 = local read "Pel"() -> (w757:dbl)
                        n4027 = local read "bin"() -> (w772:dbl)
                        n4028 = local read "Override AI buffer"() -> (w755:bool)
                        n4029 = local read "finite samples"() -> (w781:bool)
                        n4030 = local read "srateAODOtt"() -> (w768:dbl)
                        n4031 = local read "srateAODOtt"() -> (w775:dbl)
                        n4032 = local read "continuous"() -> (w780:bool)
                        n4033 = local read "Angle ref"() -> (w765:dbl)
                        n4034 = local read "wavdet"() -> (w782:bool)
                        n4035 = local read "Vx-ref"() -> (w777:dbl)
                        n4036 = local read "Vy-ref"() -> (w779:dbl)
                        n4037 = local read "avpp"() -> (w778:i32)
                        n4038 = call "tt_timeandsamples.vi"("bin"=w772, "refreshtime"=w766, "srateAODOtt"=w769, "tot#ofsamples"=w774) -> ("refreshrate"=w770:dbl, "refreshbuffer"=w771:i32, "timetracecycles"=w776:i32)  [unwired: 5 in]
                        n4039 = local read "bin"() -> (w773:dbl)
                        n4040 = call "2pparameters.vi"("command"="get") -> ("params out"=w785:T12)  [unwired: 1 in]
                        n4041 = Bundle By Name(cluster=w785, "Drawing Mode"=w758, "measpoints"=w774, "tt_cycles"=w776, "refreshbuffer"=w771, "refreshrate"=w770, "Vx-ref"=w777, "Vy-ref"=w779, "srate"=w768, "finite"=w781, "cont"=w780, "wavdet"=w782, "avpp"=w778, "srateAODO"=w775, "bufferAI"=w771, "bin"=w773, "Angle Img"=w765, "Vxminref"=w764, "Vxmaxref"=w763, "Vyminref"=w762, "Vymaxref"=w761, "Xpixels Img"=w760, "Ypixels Img"=w759, "Pel"=w757, "Vz-reset"=0.0, "AIoverride"=w755, "type"="Lifetime (contour)") -> (w783:T12)
                        n4042 = Reciprocal(x=w770) -> (1/x=w767:dbl)
                        n4043 = local write "refreshtime"(w767) -> ()
                        n4044 = call "2pparameters.vi"("Params in"=w783, "command"="set") -> ()  [unwired: 1 out]
                      }
                      frame "X-Y-Z-t movie" {
                      }
                      frame "linescan" {
                      }
                      frame "Timetrace" {
                        n4045 = local read "Vy-min draw"() -> (w795:dbl)
                        n4046 = local read "Vy-max draw"() -> (w794:dbl)
                        n4047 = local read "Vx-min draw"() -> (w797:dbl)
                        n4048 = local read "Vx-max draw"() -> (w796:dbl)
                        n4049 = local read "xpixels ref"() -> (w793:i32)
                        n4050 = local read "ypixels ref"() -> (w792:i32)
                        n4051 = local read "ROI Type"() -> (w791:u16)
                        n4052 = local read "srateAODOtt"() -> (w802:dbl)
                        n4053 = local read "# of frames"() -> (w807:i32)
                        n4054 = local read "refreshtime"() -> (w799:dbl)
                        n4055 = local read "Pel"() -> (w790:dbl)
                        n4056 = local read "bin"() -> (w805:dbl)
                        n4057 = local read "Override AI buffer"() -> (w788:bool)
                        n4058 = local read "finite samples"() -> (w814:bool)
                        n4059 = local read "srateAODOtt"() -> (w801:dbl)
                        n4060 = local read "srateAODOtt"() -> (w808:dbl)
                        n4061 = local read "continuous"() -> (w813:bool)
                        n4062 = local read "Angle ref"() -> (w798:dbl)
                        n4063 = local read "wavdet"() -> (w815:bool)
                        n4064 = local read "Vx-ref"() -> (w810:dbl)
                        n4065 = local read "Vy-ref"() -> (w812:dbl)
                        n4066 = local read "avpp"() -> (w811:i32)
                        n4067 = call "tt_timeandsamples.vi"("bin"=w805, "refreshtime"=w799, "srateAODOtt"=w802, "tot#ofsamples"=w807) -> ("refreshrate"=w803:dbl, "refreshbuffer"=w804:i32, "timetracecycles"=w809:i32)  [unwired: 5 in]
                        n4068 = local read "bin"() -> (w806:dbl)
                        n4069 = call "2pparameters.vi"("command"="get") -> ("params out"=w818:T12)  [unwired: 1 in]
                        n4070 = Bundle By Name(cluster=w818, "Drawing Mode"=w791, "measpoints"=w807, "tt_cycles"=w809, "refreshbuffer"=w804, "refreshrate"=w803, "Vx-ref"=w810, "Vy-ref"=w812, "srate"=w801, "finite"=w814, "cont"=w813, "wavdet"=w815, "avpp"=w811, "srateAODO"=w808, "bufferAI"=w804, "bin"=w806, "Angle Img"=w798, "Vxminref"=w797, "Vxmaxref"=w796, "Vyminref"=w795, "Vymaxref"=w794, "Xpixels Img"=w793, "Ypixels Img"=w792, "Pel"=w790, "Vz-reset"=0.0, "AIoverride"=w788, "type"="Timetrace") -> (w816:T12)
                        n4071 = Reciprocal(x=w803) -> (1/x=w800:dbl)
                        n4072 = local write "refreshtime"(w800) -> ()
                        n4073 = call "2pparameters.vi"("Params in"=w816, "command"="set") -> ()  [unwired: 1 out]
                      }
                      frame "Lifetime (point)" {
                      }
                    }
                  }
                  frame #1 {
                    w821 = FALSE ("wavdet")
                    n4074 = call "2pparameters.vi"("command"="get") -> ("params out"=w825:T12)  [unwired: 1 in]
                    n4075 = Bundle By Name(cluster=w825, "finite"=w821, "cont"=w821, "wavdet"=TRUE) -> (w822:T12)
                    n4076 = call "2pparameters.vi"("Params in"=w822, "command"="set") -> ()  [unwired: 1 out]
                  }
                  frame #2 {
                    n4077 = local read "DO channels"() -> (w833:u16)
                    n4078 = call "2pparameters.vi"("command"="get") -> ("params out"=w831:T12)  [unwired: 1 in]
                    n4079 = in-place {
                      in-place-border: w833 -> [w838]
                      in-place-border: [w835] -> w828
                      in-place-border: [w834] -> w827
                      n4080 = in-place-cluster #52(w831) -> ("aDO"=w837:u32[])
                      n4081 = call "remove channel from active arrayv2.vi"("line array in"=w837, "line to remove"=w838) -> ("line array out"=w836:u32[], "removal"=w835:bool, "index"=w834:i32)
                      n4082 = in-place-cluster #52("aDO"=w836) -> (w829:T12)
                    }
                    n4083 = local write "remDO"(w828) -> ()
                    n4084 = call "2pparameters.vi"("Params in"=w829, "command"="set") -> ()  [unwired: 1 out]
                  }
                  frame #3 {
                    n4085 = local read "remDO"() -> (w839:bool)
                    n4086 = case shown="True" w839 {
                      frame False {
                      }
                      frame True {
                        n4087 = call "Used AO lines.vi"() -> ("used AO names"=w843:string[], "used AO lines"=w845:tag[])  [unwired: 2 in]
                        n4088 = local write "Analog Used Lines"(w845) -> ()
                        n4089 = local write "Analog Used Names"(w843) -> ()
                        n4090 = call "Used DO lines.vi"() -> ("used DO names"=w841:string[], "used DO lines"=w840:tag[])  [unwired: 2 in]
                        n4091 = control-ref of="Analog Lines Plot"() -> (w844:refnum<vi>)
                        n4092 = control-ref of="Digital Lines Plot"() -> (w842:refnum<vi>)
                        n4093 = local write "Digital Used Lines"(w840) -> ()
                        n4094 = local write "Digital Used Names"(w841) -> ()
                        n4095 = call "prepAOWaveplot.vi"("WaveformGraph in"=w844, "Analog Used Names"=w843) -> ()  [unwired: 1 in]
                        n4096 = call "prepDOWaveplot.vi"("DigitalGraph in"=w842, "used DO names"=w841) -> ()  [unwired: 1 in]
                      }
                    }
                  }
                  frame #4 {
                    n4097 = local read "remDO"() -> (w847:bool)
                    n4098 = case shown="True" w847 {
                      tunnel: w846 -> [_ w848]
                      frame False {
                      }
                      frame True {
                        n4099 = call "waveformparamsv2.vi"("command"="rem DO", "index"=w848) -> ()  [unwired: 3 in, 3 out]
                      }
                    }
                  }
                  frame #5 {
                    n4100 = local read "Meastab"() -> (w853:enum32{"X-Y Image", "Linescan", "Timetrace"})
                    n4101 = property on="refwf" class="Ring (strict)"() -> ("RingText.Text"=w860:string)  [unwired: 2 in, 2 out]
                    n4102 = call "waveformsDObuffer.vi"("command"="get") -> ("DO wf out"=w859:digitalwaveform[])  [unwired: 1 in]
                    n4103 = case shown="\"Timetrace\"" w853 {
                      tunnel: [w869 w870] -> w852
                      frame "X-Y Image", Default {
                        n4104 = local read "Sampling rate"() -> (w869:dbl)
                      }
                      frame "Timetrace" {
                        n4105 = local read "srateAODOtt"() -> (w870:dbl)
                      }
                    }
                    n4106 = call "waveformsAObuffer.vi"("command"="get") -> ("AO wf out"=w868:waveform(dbl)[])  [unwired: 1 in]
                    n4107 = Delete From Array(array=w859, length=1, index=w857) -> (array with subset deleted=w856:digitalwaveform[])  [unwired: 1 out]
                    n4108 = call "correctwaveformsizetemp.vi"("new sampling frequency (Hz)"=w852, "start"=FALSE, "reference waveforms to"=w860, "Analog waveforms in"=w868, "stop"=FALSE, "Digital waveforms in"=w856) -> ("analog wf out"=w863:waveform(dbl)[], "Digital wf out"=w861:digitalwaveform[], "measpoints"=w854:i32)
                    n4109 = local read "wavdet"() -> (w855:bool)
                    n4110 = call "waveformsAObuffer.vi"("AO wf in"=w863, "command"="set") -> ()  [unwired: 1 out]
                    n4111 = call "waveformsDObuffer.vi"("DO wf in"=w861, "command"="set") -> ()  [unwired: 1 out]
                    n4112 = local write "Analog Lines Plot"(w863) -> ()
                    n4113 = local write "Digital Lines Plot"(w861) -> ()
                    n4114 = call "GetNumCamFramesv2.vi"("Digital Waveform Graph"=w861) -> ("Numeric"=w862:i32)  [unwired: 10 in]
                    n4115 = case shown="True" w855 {
                      tunnel: w854 -> [_ w871]
                      frame False {
                      }
                      frame True {
                        n4116 = local write "# of frames"(w871) -> ()
                      }
                    }
                    n4117 = local write "Total Camera Frames"(w862) -> ()
                  }
                  frame #6 {
                    w872 = FALSE ("addAO")
                    n4118 = local read "finite samples"() -> (w873:bool)
                    n4119 = local read "continuous"() -> (w874:bool)
                    n4120 = local read "wavdet"() -> (w875:bool)
                    n4121 = local write "remDO"(w872) -> ()
                    n4122 = call "2pparameters.vi"("command"="get") -> ("params out"=w878:T12)  [unwired: 1 in]
                    n4123 = Bundle By Name(cluster=w878, "finite"=w873, "cont"=w874, "wavdet"=w875) -> (w876:T12)
                    n4124 = property on="Rem DO wave" class="Bool (strict)"("Val(Sgnl)"=w872) -> ()  [unwired: 2 in, 2 out]
                    n4125 = call "2pparameters.vi"("Params in"=w876, "command"="set") -> ()  [unwired: 1 out]
                  }
                }
              }
            }
          }
          event "Digital phase (s)", "Digital DC (%)", "Digital Freq (Hz)", "Digital padding value", "Digital time offset (s)": Value Change {
            n4126 = event-data() -> ()  [unwired: 1 in, 6 out]
            n4127 = stacked-sequence {
              seq-local: [_ _ w986 _ _] -> [_ _ _ w1003 _]
              seq-local: [_ _ w985 _ _] -> [_ _ _ w1002 _]
              frame #0 {
                n4128 = local read "Measurement"() -> (w880:T5)
                n4129 = case shown="\"X-Y-t movie\", Default" w880 {
                  frame "X-Y-t movie", Default {
                    n4130 = local read "avpp"() -> (w901:i32)
                    n4131 = local read "Angle ref"() -> (w900:dbl)
                    n4132 = local read "ROI Type"() -> (w899:u16)
                    n4133 = local read "xpixels ref"() -> (w896:i32)
                    n4134 = local read "Vx-min ref"() -> (w895:dbl)
                    n4135 = local read "Vx-max ref"() -> (w894:dbl)
                    n4136 = local read "ypixels ref"() -> (w892:i32)
                    n4137 = local read "Vy-min ref"() -> (w893:dbl)
                    n4138 = local read "Vy-max ref"() -> (w889:dbl)
                    n4139 = local read "Sampling rate"() -> (w883:dbl)
                    n4140 = local read "finite samples"() -> (w884:bool)
                    n4141 = local read "continuous"() -> (w887:bool)
                    n4142 = local read "wavdet"() -> (w888:bool)
                    n4143 = local read "# of frames"() -> (w886:i32)
                    n4144 = local read "maxbufferAI"() -> (w885:i32)
                    n4145 = local read "Override AI buffer"() -> (w881:bool)
                    n4146 = call "2pparameters.vi"("command"="get") -> ("params out"=w898:T12)  [unwired: 1 in]
                    n4147 = Bundle By Name(cluster=w898, "type"="X-Y-t movie", "avpp"=w901, "Angle Img"=w900, "Xpixels Img"=w896, "Vx-min Img"=w895, "VX-max Img"=w894, "Ypixels Img"=w892, "Vy-min Img"=w893, "Vy-max Img"=w889, "srate"=w883, "srate Img"=w883, "finite"=w884, "cont"=w887, "wavdet"=w888, "measpoints"=w886, "maxbufferAI"=w885, "Drawing Mode"=w899, "Vz-reset"=0.0, "AIoverride"=w881) -> (w890:T12)
                    n4148 = call "2pparameters.vi"("Params in"=w890, "command"="set") -> ()  [unwired: 1 out]
                  }
                  frame "X-Y-Z stack" {
                    n4149 = call "2pparameters.vi"("command"="get") -> ("params out"=w905:T12)  [unwired: 1 in]
                    n4150 = Bundle By Name(cluster=w905, "type"="X-Y-Z stack") -> (w903:T12)
                    n4151 = call "2pparameters.vi"("Params in"=w903, "command"="set") -> ()  [unwired: 1 out]
                  }
                  frame "Lifetime (scan)" {
                    n4152 = call "2pparameters.vi"("command"="get") -> ("params out"=w910:T12)  [unwired: 1 in]
                    n4153 = Bundle By Name(cluster=w910, "type"="Lifetime (scan)") -> (w908:T12)
                    n4154 = call "2pparameters.vi"("Params in"=w908, "command"="set") -> ()  [unwired: 1 out]
                  }
                  frame "Lifetime (contour)" {
                    n4155 = local read "Vy-min draw"() -> (w920:dbl)
                    n4156 = local read "Vy-max draw"() -> (w919:dbl)
                    n4157 = local read "Vx-min draw"() -> (w922:dbl)
                    n4158 = local read "Vx-max draw"() -> (w921:dbl)
                    n4159 = local read "xpixels ref"() -> (w918:i32)
                    n4160 = local read "ypixels ref"() -> (w917:i32)
                    n4161 = local read "ROI Type"() -> (w916:u16)
                    n4162 = local read "srateAODOtt"() -> (w927:dbl)
                    n4163 = local read "# of frames"() -> (w932:i32)
                    n4164 = local read "refreshtime"() -> (w924:dbl)
                    n4165 = local read "Pel"() -> (w915:dbl)
                    n4166 = local read "bin"() -> (w930:dbl)
                    n4167 = local read "Override AI buffer"() -> (w913:bool)
                    n4168 = local read "finite samples"() -> (w939:bool)
                    n4169 = local read "srateAODOtt"() -> (w926:dbl)
                    n4170 = local read "srateAODOtt"() -> (w933:dbl)
                    n4171 = local read "continuous"() -> (w938:bool)
                    n4172 = local read "Angle ref"() -> (w923:dbl)
                    n4173 = local read "wavdet"() -> (w940:bool)
                    n4174 = local read "Vx-ref"() -> (w935:dbl)
                    n4175 = local read "Vy-ref"() -> (w937:dbl)
                    n4176 = local read "avpp"() -> (w936:i32)
                    n4177 = call "tt_timeandsamples.vi"("bin"=w930, "refreshtime"=w924, "srateAODOtt"=w927, "tot#ofsamples"=w932) -> ("refreshrate"=w928:dbl, "refreshbuffer"=w929:i32, "timetracecycles"=w934:i32)  [unwired: 5 in]
                    n4178 = local read "bin"() -> (w931:dbl)
